vi "Execute.vi"(6 "Error":errorcluster, 7 "Actor":refnum<class "Actor.lvclass">, 10 "Msg":T1, 11 "Actor":T2) -> (3 "Actor":T2, 4 "Error":errorcluster, 5 "Actor":refnum<class "Actor.lvclass">)   [LabVIEW 2020, in "jettl.lvlib"]
uses:
  jettl.lvlib
  Actor/Actor.lvclass
  Msg/Msg.lvclass
  Origin.ctl
  Metadata/Metadata.lvclass
  Lifecycle.ctl
  MsgExecuteType.ctl
  MsgAttribs.ctl
  Msg.ctl
  PostSetup.ctl
  PreSetup.ctl
  MsgNames.ctl
  ActorAttribs.ctl
  ChildActors.ctl
  Actor.ctl
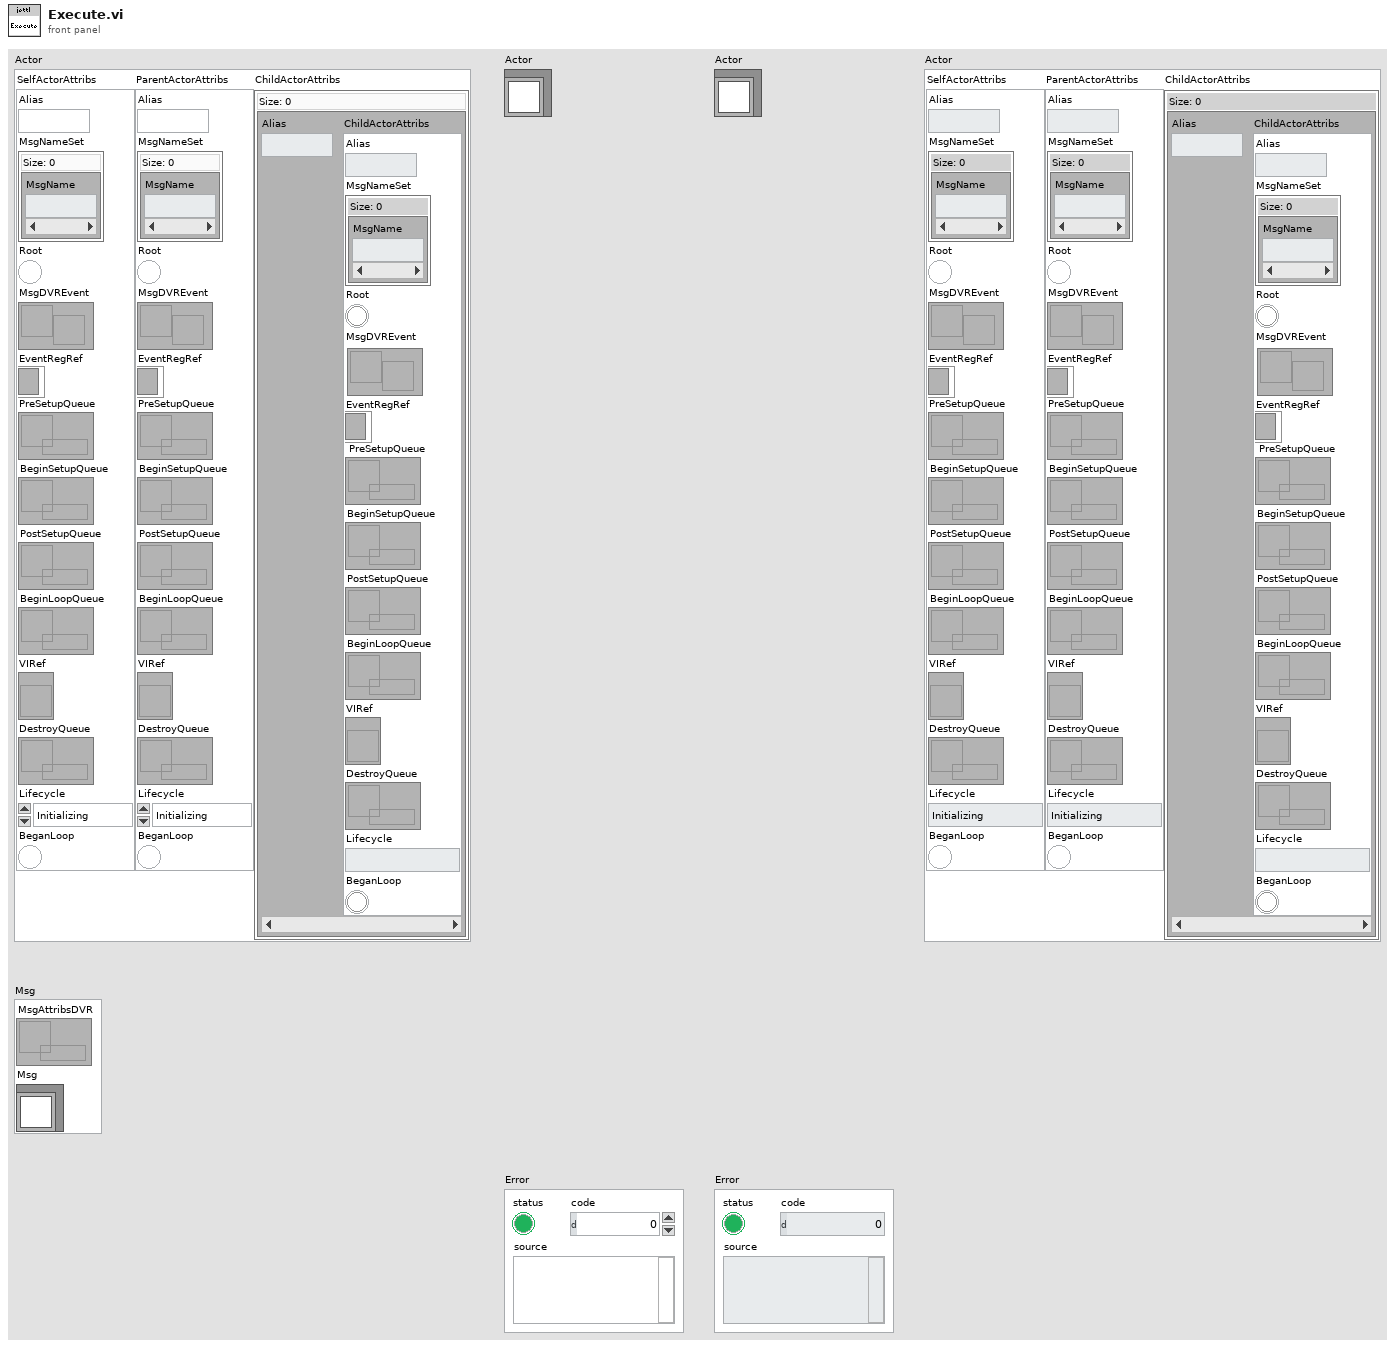
[diagram p1: front panel]
types:
  T1 = typedef "jettl.lvlib/Msg.ctl" = cluster{"MsgAttribsDVR":refnum<data-value>, "Msg":refnum<class "Msg.lvclass">}
  T2 = typedef "jettl.lvlib/Actor.ctl" = cluster{"SelfActorAttribs":T3, "ParentActorAttribs":T3, "ChildActorAttribs":T6}
  T3 = typedef "jettl.lvlib/ActorAttribs.ctl" = cluster{"Alias":string, "MsgNameSet":T4, "Root":bool, "MsgDVREvent":refnum<user-event>, "EventRegRef":refnum<event-registration>, "PreSetupQueue":refnum<queue>, "BeginSetupQueue":refnum<queue>, "PostSetupQueue":refnum<queue>, "BeginLoopQueue":refnum<queue>, "VIRef":refnum<vi>, "DestroyQueue":refnum<queue>, "Lifecycle":T5, "BeganLoop":bool}
  T4 = typedef "jettl.lvlib/MsgNames.ctl" = set{string}
  T5 = typedef "jettl.lvlib/Lifecycle.ctl" = enum16{"Initializing", "SettingUp", "Starting", "Running", "Stopping", "TearingDown", "Terminated"}
  T6 = typedef "jettl.lvlib/ChildActors.ctl" = map{string, T3}
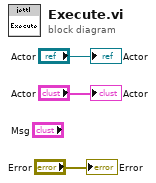
[diagram p0: block diagram]
diagram:
  "Actor" <- "Actor"
  "Actor" <- "Actor"
  "Error" <- "Error"
